vi "Error Query.vi"(8 "error in (no error)":errorcluster, 11 "VISA resource name":refnum<visa-resource-name>) -> (0 "error out":errorcluster, 2 "Error Message":string, 3 "VISA resource name out":refnum<visa-resource-name>)   [LabVIEW 2020, in "Stanford Research SR865.lvlib"]
doc: "Queries the instrument for any errors in the instrument's error queue. It will continue to read errors until all errors have been read from the instrument. Any errors will be returned in the <B>error out</B> control.\n\n<B>Note:</B>\nThis VI is called automatically by most driver VIs so it is not usually necessary to call this in an application."
uses:
  Stanford Research SR865.lvlib
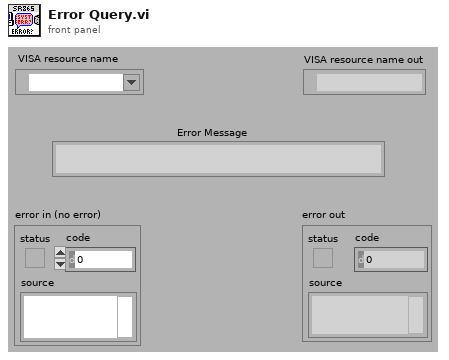
[diagram p1: front panel]
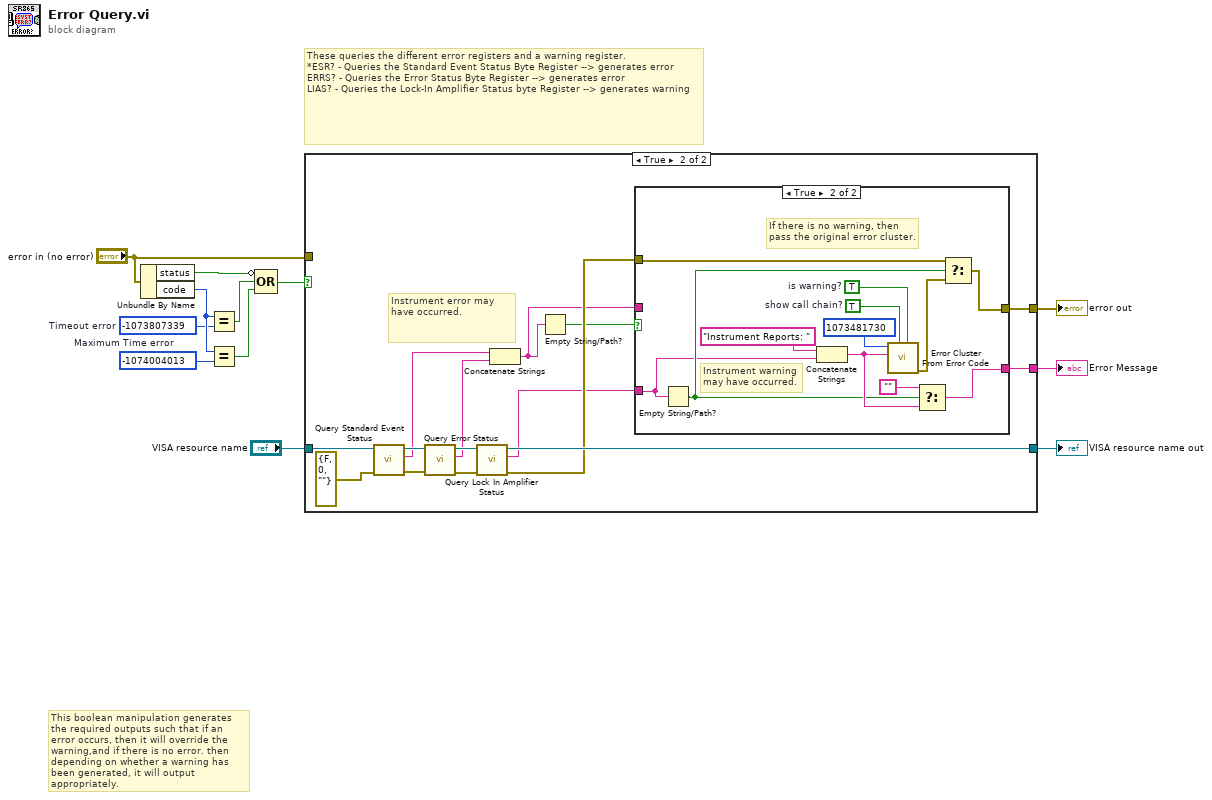
[diagram p0: block diagram]
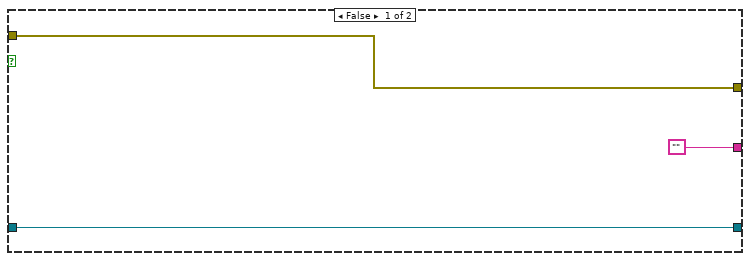
[diagram p2: hidden frame]
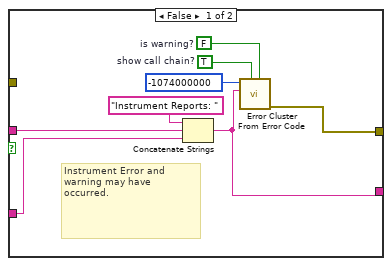
[diagram p3: hidden frame]
diagram:
  w10 = -1074004013  # Maximum Time error
  w2 = -1073807339  # Timeout error
  # "This boolean manipulation generates the required outputs such that if an error occurs, then it will override the warning,and if there is no error. then depending on whether a warning has been generated, it will output appropriately."
  # "These queries the different error registers and a warning register. \n*ESR? - Queries the Standard Event Status Byte Register --> generates error\nERRS? - Queries the Error Status Byte Register --> generates error\nLIAS? - Queries the Lock-In Amplifier Status byte Register --> generates warning"
  n1 = Unbundle By Name("error in (no error)") -> ("status"=w1:bool, "code"=w11:i32)
  n2 = Equal?(x=w11, y=w2) -> (x = y?=w3:bool)
  n3 = Equal?(x=w11, y=w10) -> (x = y?=w12:bool)
  n4 = Compound Arithmetic op=OR(invert w1, w3, w12) -> (w4:bool)
  n5 = case shown="True" w4 {
    tunnel: "VISA resource name" -> [w15 w30]
    tunnel: "error in (no error)" -> [w14 _]
    tunnel: ["" w23] -> w7
    tunnel: [w14 w25] -> w8
    tunnel: [w15 w26] -> w9
    frame False {
    }
    frame True {
      # "Instrument error may have occurred."
      n6 = call "Query Standard Event Status.vi"("error in (no error)"=errorcluster {"status"=FALSE, "code"=0, "source"=""}, "VISA resource name"=w30) -> ("error out"=w22:errorcluster, "Standard Event Status Data Message"=w20:string, "VISA resource name out"=w29:refnum<visa-resource-name>)  [unwired: 7 in]
      n7 = call "Query Error Status.vi"("error in (no error)"=w22, "VISA resource name"=w29) -> ("error out"=w21:errorcluster, "Error Status Data Message"=w19:string, "VISA resource name out"=w27:refnum<visa-resource-name>)  [unwired: 7 in]
      n8 = call "Query Lock In Amplifier Status.vi"("error in (no error)"=w21, "VISA resource name"=w27) -> ("error out"=w24:errorcluster, "Lock In Amplifier Data Message"=w18:string, "VISA resource name out"=w26:refnum<visa-resource-name>)  [unwired: 7 in]
      n9 = Concatenate Strings(w20, w19) -> (w17:string)
      n10 = Empty String/Path?(string/path=w17) -> (empty?=w16:bool)
      n11 = case shown="True" w16 {
        tunnel: [w35 w47] -> w25
        tunnel: w24 -> [_ w41]
        tunnel: [w34 w46] -> w23
        tunnel: w17 -> [w32 _]
        tunnel: w18 -> [w31 w39]
        frame False {
          w36 = FALSE  # is warning?
          w37 = TRUE  # show call chain?
          # "Instrument Error and warning may have occurred."
          n12 = Concatenate Strings("Instrument Reports: " ("string"), w32, w31) -> (w34:string)
          n13 = call <vilib>:"Error Cluster From Error Code.vi"("is warning? (False)"=w36, "show call chain? (False)"=w37, "error message (\"\")"=w34, "error code (0)"=-1074000000 ("t")) -> ("error out"=w35:errorcluster)  [unwired: 5 in]
        }
        frame True {
          w48 = TRUE  # is warning?
          w49 = TRUE  # show call chain?
          # "If there is no warning, then pass the original error cluster."
          # "Instrument warning may have occurred."
          n14 = Empty String/Path?(string/path=w39) -> (empty?=w40:bool)
          n15 = Concatenate Strings("Instrument Reports: " ("string"), w39) -> (w43:string)
          n16 = call <vilib>:"Error Cluster From Error Code.vi"("is warning? (False)"=w48, "show call chain? (False)"=w49, "error message (\"\")"=w43, "error code (0)"=1073481730 ("t")) -> ("error out"=w42:errorcluster)  [unwired: 5 in]
          n17 = Select(t="" ("f"), s=w40, f=w43) -> (s? t:f=w46:string)
          n18 = Select(t=w41, s=w40, f=w42) -> (s? t:f=w47:errorcluster)
        }
      }
    }
  }
  "error out" <- w8
  "VISA resource name out" <- w9
  "Error Message" <- w7
